vi "VisualizeBase.vi"() -> ()   [LabVIEW 2014, in "Visualization.lvlib" / "VisualizeBase.lvclass"]
uses:
  VisualizeBase.lvclass
  Requests/clUserEventType.ctl
  <vilib>/event_ctls.llb/usereventprio.ctl
  <vilib>/Utility/error.llb/Error Cluster From Error Code.vi
  <vilib>/ErrorRing/Error Ring.xnode
  <userlib>/NIST/NISTErrorLib/NISTErrorLib.lvlib
panel:
  in  "QueName":string="BaseVisQue"
  out "ErrorArray":errorcluster[](array[cluster])
  in  "btnStop":bool
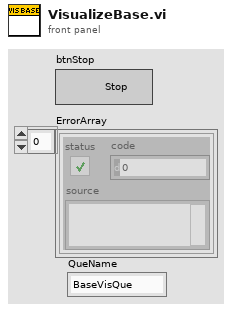
[diagram p1: front panel]
types:
  T1 = typedef "Visualization.lvlib/VisualizeBase.lvclass/clRequestEvents.ctl" = cluster{"StopRequest":refnum<user-event>}
  T2 = typedef "Visualization.lvlib/VisualizeBase.lvclass/clUserEventType.ctl" = cluster{"BusIndex":i8, "Data":variant}
  T3 = typedef "usereventprio.ctl" = enum32{"high priority", "normal priority"}
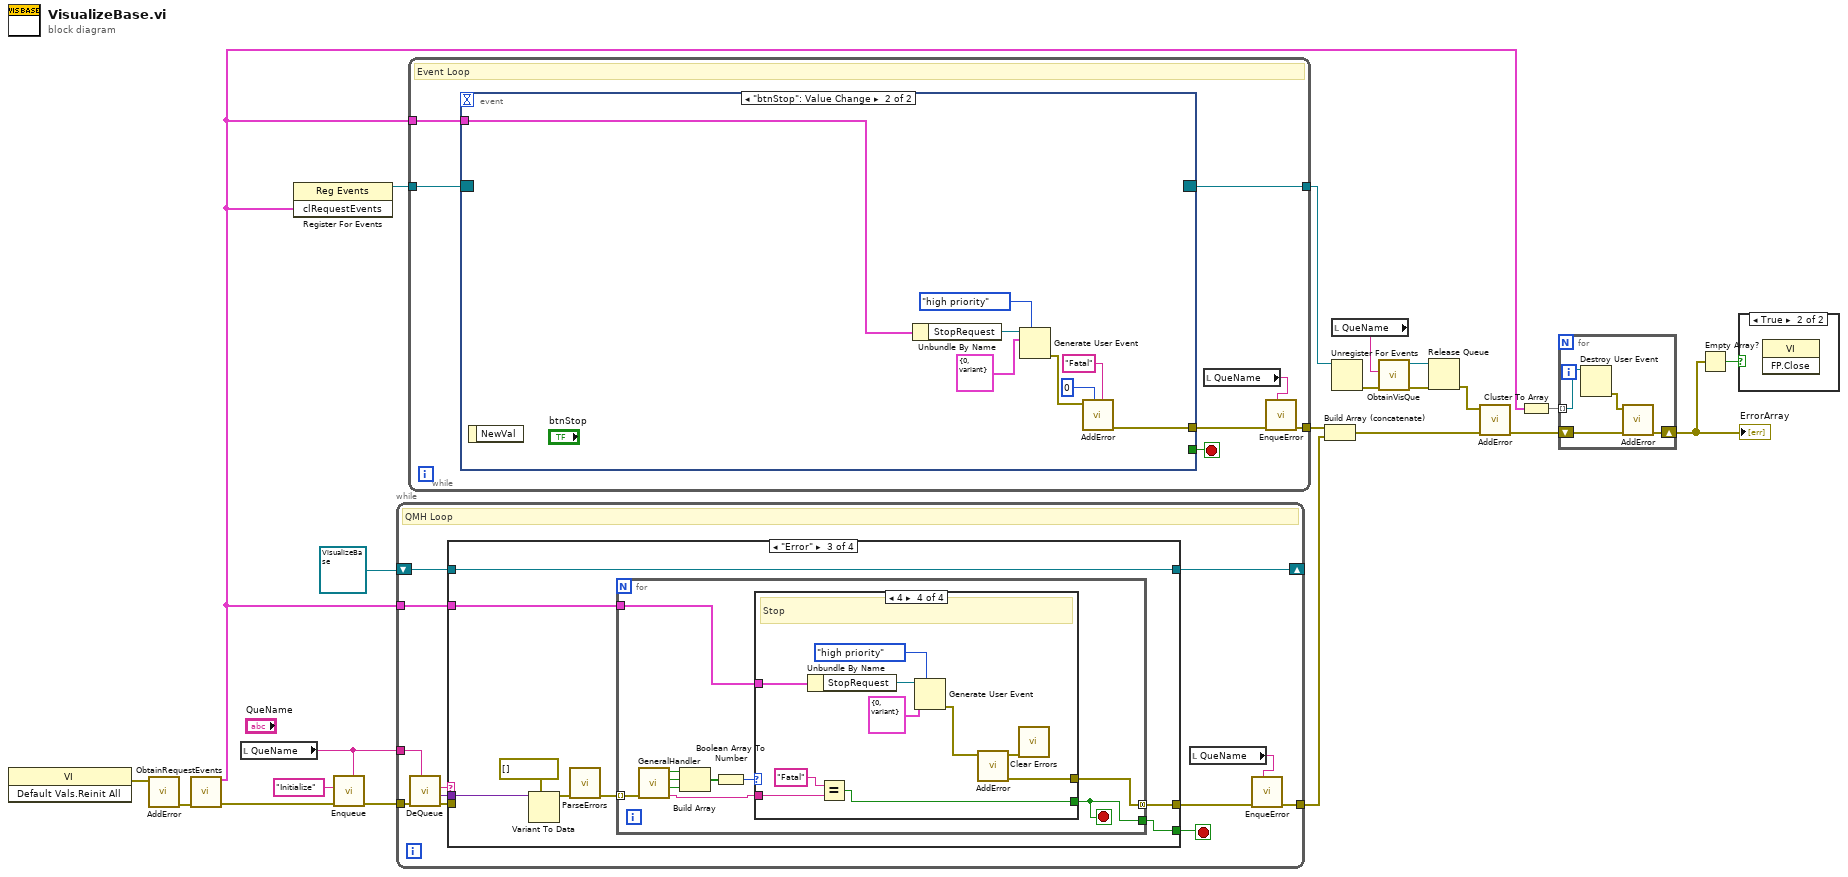
[diagram p0: block diagram]
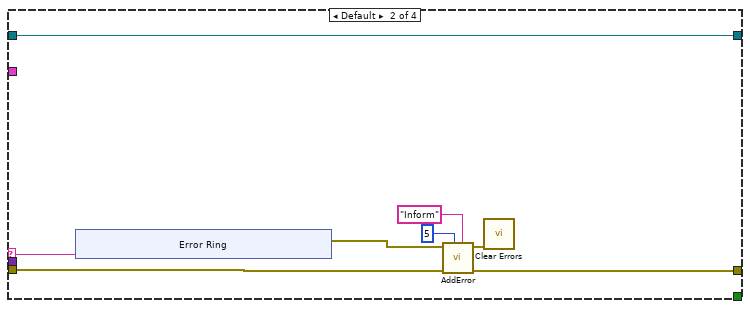
[diagram p4: hidden frame]
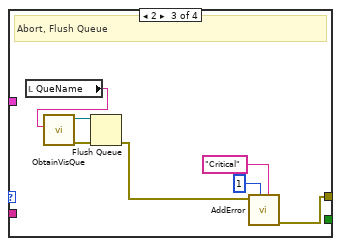
[diagram p7: hidden frame]
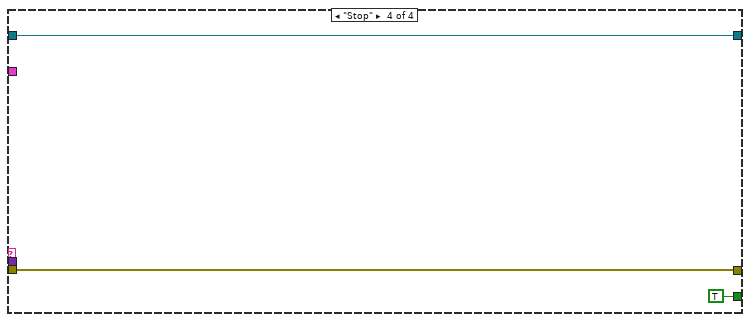
[diagram p8: hidden frame]
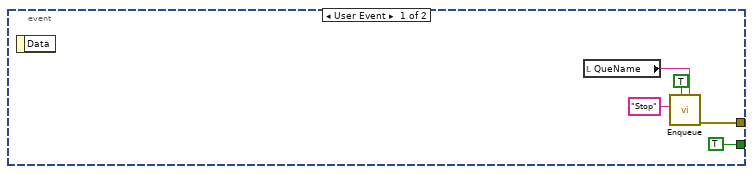
[diagram p9: hidden frame]
diagram:
  n1 = invoke class="VI" method="Default Vals.Reinit All"() -> (error out=w19:errorcluster)  [unwired: 3 in, 2 out]
  n2 = call <userlib>:"AddError.vi"("error in (no error)"=w19) -> ("ErrorArray"=w18:errorcluster[])  [unwired: 9 in, 1 out]
  n3 = call "ObtainRequestEvents.vi"("Error"=w18) -> ("Error"=w16:errorcluster[], "clRequestEvents"=w3:T1)  [unwired: 9 in]
  n4 = local read "QueName"() -> (w17:string)
  n5 = register-events(w3) -> (reference out=w20:refnum<event-registration>)  [unwired: 2 in, 1 out]
  n6 = call "Enqueue.vi"("QueName"=w17, "Error"=w16, "Message"="Initialize") -> ("Error"=w21:errorcluster[])  [unwired: 8 in]
  n7 = while {
    tunnel: w21 -> [w34]
    tunnel: [w28] -> w11
    tunnel: w17 -> [w26]
    shift-right: [w25] -> _
    shift-left: refnum<class "VisualizeBase.lvclass"> refnum ("VisualizeBase_class.lvclass") -> [w24]
    tunnel: w3 -> [w23]
    stop <- w29 stop-if-true
    # "QMH Loop"
    n8 = call "DeQueue.vi"("QueName"=w26, "Error"=w34) -> ("Error"=w31:errorcluster[], "Data"=w32:variant, "Message"=w33:string)  [unwired: 7 in]
    n9 = case shown="\"Error\"" w33 {
      selector: w33 -> [_ w44 _ _]
      tunnel: w32 -> [_ _ w59 _]
      tunnel: w31 -> [w36 w42 _ w88]
      tunnel: [w36 w41 w55 w88] -> w30
      tunnel: [_ _ w54 TRUE] -> w29
      tunnel: w24 -> [w35 w37 w53 w87]
      tunnel: [w35 w37 w53 w87] -> w25
      tunnel: w23 -> [_ _ w52 _]
      frame "Initialize" {
      }
      frame Default {
        n10 = xnode "Error Ring"("parameter 0"=w44) -> ("error out"=w43:errorcluster)
        n11 = call <userlib>:"AddError.vi"("Severity"="Inform" ("String"), "Priority"=u8 5, "ErrorArray"=w42, "error in (no error)"=w43) -> ("ErrorArray"=w41:errorcluster[], "error out"=w40:errorcluster)  [unwired: 6 in]
        n12 = call <vilib>:"Clear Errors.vi"("error in (no error)"=w40) -> ()  [unwired: 5 in, 2 out]
      }
      frame "Error" {
        n13 = Variant To Data(type=errorcluster[] [], Variant=w59) -> (data=w57:errorcluster[])  [unwired: 1 in, 1 out]
        n14 = call <userlib>:"ParseErrors.vi"("ErrorArray"=w57) -> ("ErrorArray"=w56:errorcluster[])  [unwired: 8 in, 2 out]
        n15 = for {
          tunnel: w56 -> [w69] mode=indexing
          tunnel: [w63] -> w55 mode=concatenating
          tunnel: [w61] -> w54
          tunnel: w52 -> [w60]
          stop <- w61 stop-if-true
          n16 = call <userlib>:"GeneralHandler.vi"("error in (no error)"=w69) -> ("Severity"=w62:string, "Stop"=w66:bool, "Abort"=w67:bool, "Continue"=w68:bool)  [unwired: 7 in]
          n17 = Build Array(w68, w67, w66) -> (w65:bool[])
          n18 = Boolean Array To Number(Boolean array=w65) -> (number=w64:u32)
          n19 = case shown="4" w64 {
            tunnel: [_ _ w74 w85] -> w63
            tunnel: w62 -> [_ _ _ w80]
            tunnel: [_ _ _ w78] -> w61
            tunnel: w60 -> [_ _ _ w77]
            frame 0, Default {
              # "No Dialog"
            }
            frame 1 {
              # "Continue"
            }
            frame 2 {
              # "Abort, Flush Queue"
              n20 = local read "QueName"() -> (w70:string)
              n21 = call "ObtainVisQue.vi"("QueName"=w70) -> ("error out"=w76:errorcluster, "queue out"=w75:refnum<queue>)  [unwired: 9 in]
              n22 = Flush Queue(queue=w75, error in (no error)=w76) -> (error out=w73:errorcluster)  [unwired: 2 out]
              n23 = call <userlib>:"AddError.vi"("Severity"="Critical" ("String"), "Priority"=u8 1, "error in (no error)"=w73) -> ("ErrorArray"=w74:errorcluster[])  [unwired: 7 in, 1 out]
            }
            frame 4 {
              # "Stop"
              n24 = Unbundle By Name(w77) -> ("StopRequest"=w86:refnum<user-event>)
              n25 = Equal?(x="Fatal", y=w80) -> (x = y?=w78:bool)
              n26 = Generate User Event(priority (normal)=usereventprio."high priority", user event=w86, event data cluster=T2 {"BusIndex"=0, "Data"=variant} ("event data")) -> (error out=w84:errorcluster)  [unwired: 1 in, 1 out]
              n27 = call <userlib>:"AddError.vi"("error in (no error)"=w84) -> ("ErrorArray"=w85:errorcluster[], "error out"=w81:errorcluster)  [unwired: 9 in]
              n28 = call <vilib>:"Clear Errors.vi"("error in (no error)"=w81) -> ()  [unwired: 5 in, 2 out]
            }
          }
        }
      }
      frame "Stop" {
      }
    }
    n29 = local read "QueName"() -> (w27:string)
    n30 = call "EnqueError.vi"("QueName"=w27, "Error"=w30) -> ("Error"=w28:errorcluster[])  [unwired: 9 in]
  }
  n31 = while {
    tunnel: w20 -> [w96]
    tunnel: [w93] -> w12
    tunnel: [w91] -> w14
    tunnel: w3 -> [w90]
    stop <- w95 stop-if-true
    # "Event Loop"
    n32 = event shown="[1] \"btnStop\": Value Change" {
      selector: w96 -> [_ _]
      dyn-events: [_ _] -> w91
      timeout: _ -> [_ _]
      tunnel: [TRUE _] -> w95
      tunnel: [w100 w107] -> w94
      tunnel: w90 -> [_ w102]
      event User Event {
        n33 = event-data() -> ()  [unwired: 1 in, 1 out]
        n34 = local read "QueName"() -> (w97:string)
        n35 = call "Enqueue.vi"("QueName"=w97, "Priority? (F)"=TRUE, "Message"="Stop") -> ("Error"=w100:errorcluster[])  [unwired: 8 in]
      }
      event "btnStop": Value Change {
        n36 = event-data() -> ()  [unwired: 1 in, 1 out]
        n37 = Unbundle By Name(w102) -> ("StopRequest"=w108:refnum<user-event>)
        n38 = Generate User Event(priority (normal)=usereventprio."high priority", user event=w108, event data cluster=T2 {"BusIndex"=0, "Data"=variant} ("event data")) -> (error out=w109:errorcluster)  [unwired: 1 in, 1 out]
        n39 = call <userlib>:"AddError.vi"("Severity"="Fatal" ("String"), "Priority"=u8 0, "error in (no error)"=w109) -> ("ErrorArray"=w107:errorcluster[])  [unwired: 7 in, 1 out]
      }
    }
    n40 = local read "QueName"() -> (w92:string)
    n41 = call "EnqueError.vi"("QueName"=w92, "Error"=w94) -> ("Error"=w93:errorcluster[])  [unwired: 9 in]
  }
  n42 = Build Array (concatenate)(w12, w11) -> (w8:errorcluster[])
  n43 = local read "QueName"() -> (w9:string)
  n44 = Unregister For Events(event registration refnum=w14) -> (error out=w10:errorcluster)  [unwired: 1 in]
  n45 = call "ObtainVisQue.vi"("error in (no error)"=w10, "QueName"=w9) -> ("error out"=w7:errorcluster, "queue out"=w6:refnum<queue>)  [unwired: 8 in]
  n46 = Release Queue(queue=w6, error in (no error)=w7) -> (error out=w5:errorcluster)  [unwired: 1 in, 2 out]
  n47 = call <userlib>:"AddError.vi"("ErrorArray"=w8, "error in (no error)"=w5) -> ("ErrorArray"=w4:errorcluster[])  [unwired: 8 in, 1 out]
  n48 = Cluster To Array(cluster=w3) -> (array=w13:refnum<user-event>[])
  n49 = for {
    tunnel: w13 -> [w113] mode=indexing
    shift-right: [w112] -> w2
    shift-left: w4 -> [w111]
    n50 = Destroy User Event(user event=w113) -> (error out=w110:errorcluster)  [unwired: 1 in]
    n51 = call <userlib>:"AddError.vi"("ErrorArray"=w111, "error in (no error)"=w110) -> ("ErrorArray"=w112:errorcluster[])  [unwired: 8 in, 1 out]
  }
  "ErrorArray" <- w2
  n52 = Empty Array?(array=w2) -> (empty?=w1:bool)
  n53 = case shown="True" w1 {
    frame False {
    }
    frame True {
      n54 = invoke class="VI" method="FP.Close"() -> ()  [unwired: 3 in, 3 out]
    }
  }
